vi "IMAQ FPGA Image Transfer to Target U8.vi"(6 "Image Transfer Size Alignment":u32(ring)=1 items=["1 Pixel"=1, "8 Pixels"=8], 7 "Write Timeout (ms)":i32=5000, 8 "error in (no error)":errorcluster, 9 "DMA FIFO Reference In":refnum<k20>, 10 "Maximum Pixels per Write":i32=-1, 11 "Image":T1) -> (0 "error out":errorcluster, 1 "DMA FIFO Reference Out":refnum<k20>, 3 "Image Out":T1)   [LabVIEW 2020, in "NI_VDM_FPGA_Basics.lvlib"]
doc: "Transfers an image from the host processor to the target FPGA via a DMA FIFO."
uses:
  <vilib>/visionFPGA/NI_VDM_FPGA_Basics.lvlib
  <vilib>/vision/Image Controls.llb/IMAQ Image.ctl
  <vilib>/rvi/errors/niLvFpgaAdjustHostInterfaceError.vi
  <vilib>/rvi/interface/nirviMethod/nirviMethod.xnode
  <vilib>/vision/EDVR.llb/IMAQ ImageToEDVR 2D U8.vi
  <vilib>/rvi/errors/niLvFpgaMergeErrorWithErrorCode.vi
  <vilib>/FPGAPlugInAG/Dynamic/niLvFpga_AcquireWriteRegionFifo_Dynamic.vi
  <vilib>/FPGAPlugInAG/Dynamic/niLvFpga_WriteFifo_Dynamic.vi
  nivissvc.dll
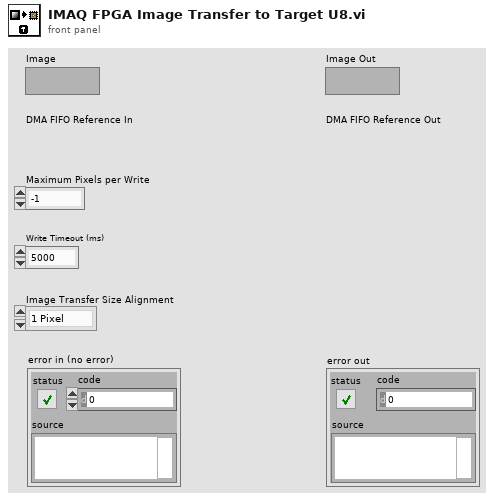
[diagram p1: front panel]
types:
  T1 = typedef "IMAQ Image.ctl" = refnum<image>
  T2 = typedef "Image Type" = u32
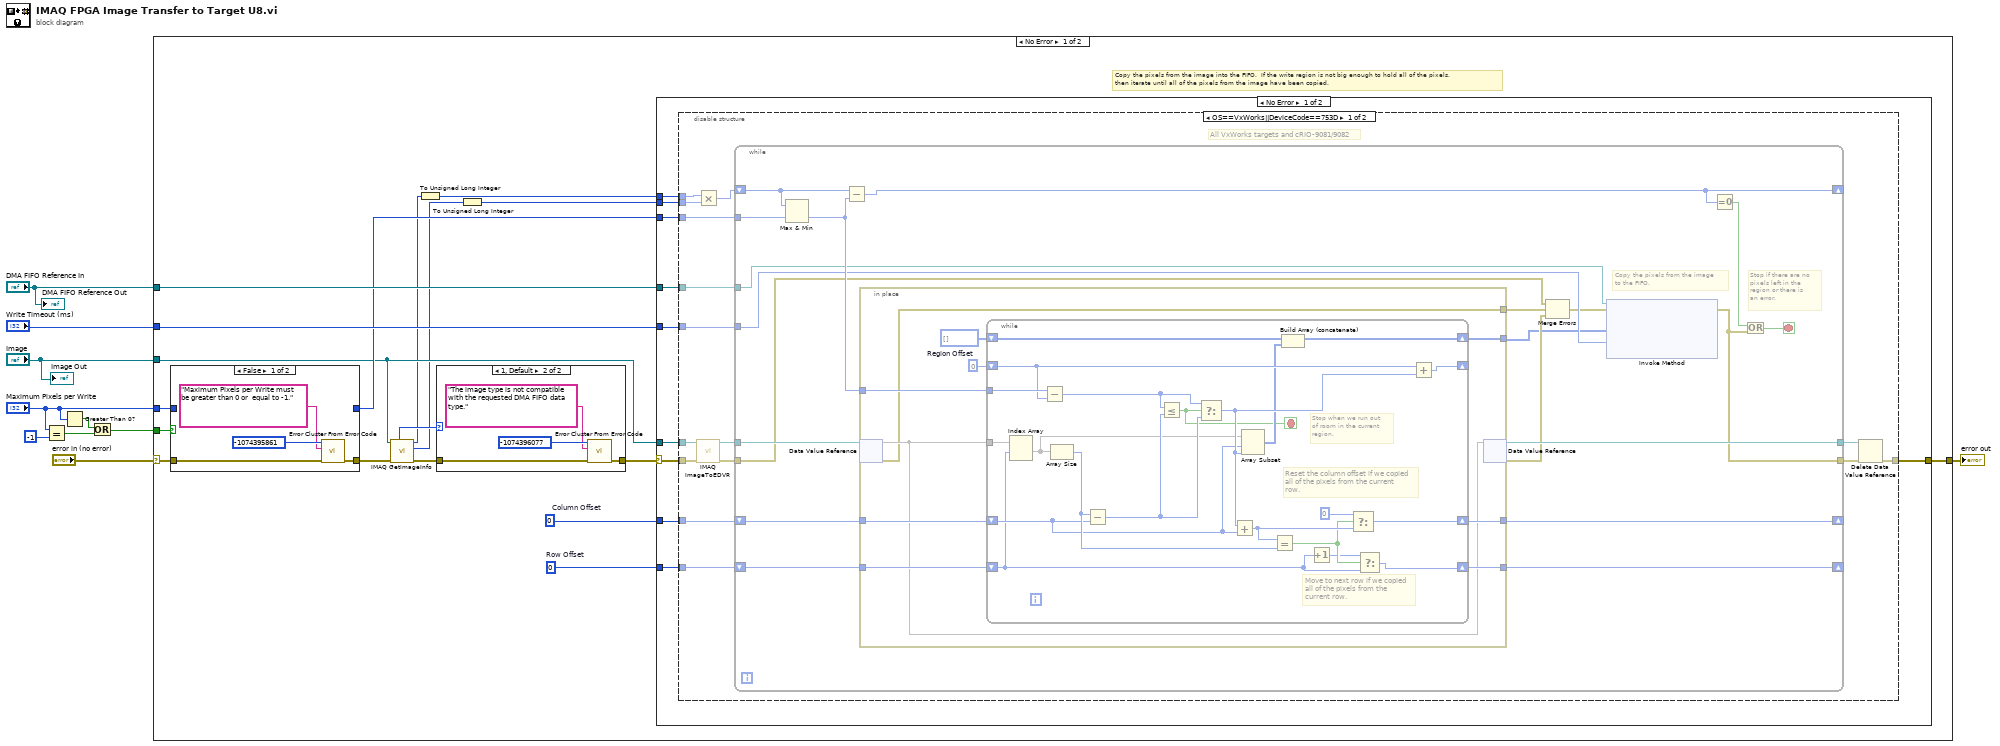
[diagram p0: block diagram]
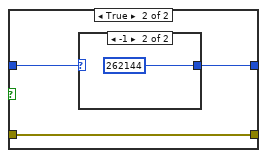
[diagram p2: hidden frame]
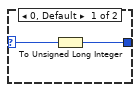
[diagram p3: hidden frame]
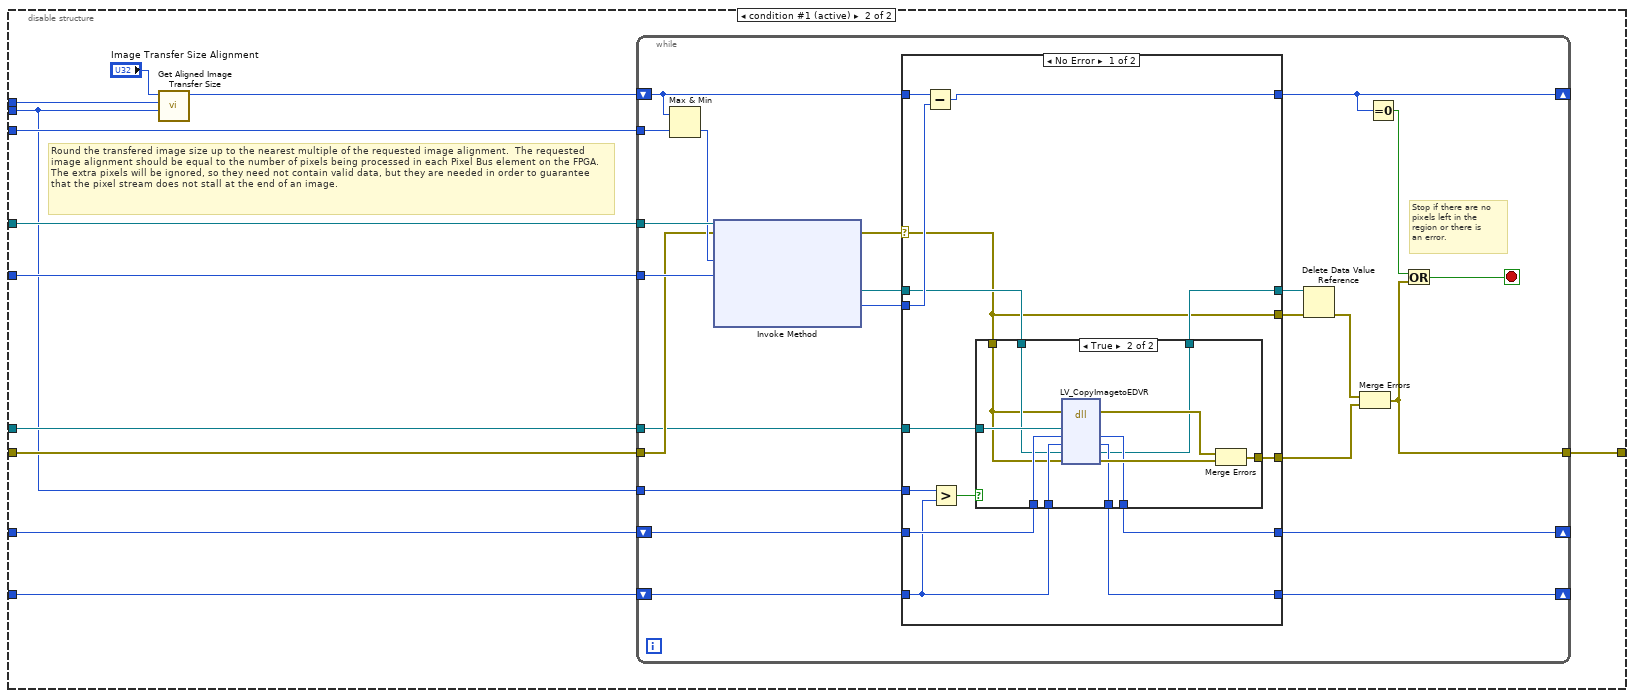
[diagram p4: hidden frame]
diagram:
  n1 = Equal?(x="Maximum Pixels per Write", y=-1) -> (x = y?=w6:bool)
  n2 = Greater Than 0?(x="Maximum Pixels per Write") -> (x > 0?=w7:bool)
  n3 = Or(x=w7, y=w6) -> (x .or. y?=w5:bool)
  n4 = case shown="No Error" "error in (no error)" {
    selector: "error in (no error)" -> [w15 w190]
    tunnel: "DMA FIFO Reference In" -> [w26 _]
    tunnel: "Write Timeout (ms)" -> [w25 _]
    tunnel: w5 -> [w22 _]
    tunnel: "Maximum Pixels per Write" -> [w19 _]
    tunnel: "Image" -> [w17 _]
    tunnel: [w16 w190] -> w2
    frame No Error {
      w23 = u32 0  # Row Offset
      w24 = u32 0  # Column Offset
      # "Copy the pixels from the image into the FIFO.  If the write region is not big enough to hold all of the pixels,\nthen iterate until all of the pixels from the image have been copied."
      n5 = case shown="False" w22 {
        tunnel: w15 -> [w30 w35]
        tunnel: [w29 w35] -> w21
        tunnel: w19 -> [_ w34]
        tunnel: [_ w33] -> w20
        frame False {
          n6 = call <vilib>:"Error Cluster From Error Code.vi"("error in (no error)"=w30, "error message (\"\")"="Maximum Pixels per Write must be greater than 0 or  equal to -1." ("error message (\"\")"), "error code (0)"=-1074395861) -> ("error out"=w29:errorcluster)  [unwired: 6 in]
        }
        frame True {
          n7 = case shown="-1" w34 {
            selector: w34 -> [w37 _]
            tunnel: [w36 u32 262144 ("Maximum Pixels per Write")] -> w33
            frame 0, Default {
              n8 = To Unsigned Long Integer(number=w37) -> (unsigned 32bit integer=w36:u32)
            }
            frame -1 {
            }
          }
        }
      }
      n9 = call "IMAQ GetImageInfo"("error in (no error)"=w21, "Image"=w17) -> ("error out"=w27:errorcluster, "Y Resolution"=w13:i32, "X Resolution"=w14:i32, "Image Type"=w28:T2)  [unwired: 2 in, 4 out]
      n10 = To Unsigned Long Integer(number=w14) -> (unsigned 32bit integer=w12:u32)
      n11 = case shown="1, Default" w28 {
        tunnel: w27 -> [w185 w187]
        tunnel: [w185 w186] -> w18
        frame 0 {
          # "Allowed types are:\nGrayscale (U8)"
        }
        frame 1, Default {
          n12 = call <vilib>:"Error Cluster From Error Code.vi"("error in (no error)"=w187, "error message (\"\")"="The image type is not compatible with the requested DMA FIFO data type." ("error message (\"\")"), "error code (0)"=-1074396077) -> ("error out"=w186:errorcluster)  [unwired: 6 in]
        }
      }
      n13 = To Unsigned Long Integer(number=w13) -> (unsigned 32bit integer=w11:u32)
      n14 = case shown="No Error" w18 {
        selector: w18 -> [w43 w184]
        tunnel: w24 -> [w45 _]
        tunnel: w23 -> [w44 _]
        tunnel: w26 -> [w47 _]
        tunnel: [w41 w184] -> w16
        tunnel: w20 -> [w48 _]
        tunnel: w25 -> [w46 _]
        tunnel: w17 -> [w42 _]
        tunnel: w12 -> [w40 _]
        tunnel: w11 -> [w39 _]
        frame No Error {
          n15 = disable-structure shown="OS==VxWorks||DeviceCode==753D" {
            disable-tunnel: w45 -> [w63 w126]
            disable-tunnel: w44 -> [w62 w125]
            disable-tunnel: w47 -> [w61 w124]
            disable-tunnel: [w52 w123] -> w41
            disable-tunnel: w48 -> [w60 w122]
            disable-tunnel: w46 -> [w59 w121]
            disable-tunnel: w43 -> [w57 w120]
            disable-tunnel: w42 -> [w58 w119]
            disable-tunnel: w40 -> [w51 w116]
            disable-tunnel: w39 -> [w50 w115]
            frame condition #0 {
              # "All VxWorks targets and cRIO-9081/9082"
              n16 = call-poly <vilib>:"IMAQ ImageToEDVR.vi"("error in (no error)"=w57, "Image"=w58) -> ("error out"=w55:errorcluster, "EDVR 2D U8"=w56:refnum<data-value>)  [unwired: 7 in, 1 out]
              n17 = Multiply(x=w51, y=w50) -> (x*y=w49:u32)
              n18 = while {
                shift-right: [w77] -> _
                shift-left: w49 -> [w74]
                tunnel: w56 -> [w83]
                shift-right: [w79] -> _
                shift-left: w63 -> [w81]
                shift-right: [w82] -> _
                shift-left: w62 -> [w80]
                tunnel: w61 -> [w68]
                tunnel: [w78] -> w54
                tunnel: [w66] -> w53
                tunnel: w60 -> [w73]
                tunnel: w59 -> [w69]
                tunnel: w55 -> [w64]
                stop <- w76 stop-if-true
                # "Copy the pixels from the image\nto the FIFO."
                # "Stop if there are no\npixels left in the \nregion or there is\nan error."
                n19 = Max & Min(x=w74, y=w73) -> (min(x,y)=w72:u32)  [unwired: 1 out]
                n20 = Subtract(x=w74, y=w72) -> (x-y=w77:u32)
                n21 = in-place {
                  in-place-border: w72 -> [w91]
                  in-place-border: [w93] -> w82
                  in-place-border: w81 -> [w90]
                  in-place-border: w80 -> [w88]
                  in-place-border: [w89] -> w79
                  in-place-border: [w85] -> w71
                  in-place-border: [w84] -> w65
                  w92 = u32 0  # Region Offset
                  n22 = in-place-dvr #1(w83) -> (w87:u8[][], w85:errorcluster)
                  n23 = while {
                    tunnel: w87 -> [w100]
                    shift-right: [w112] -> _
                    shift-left: w92 -> [w111]
                    tunnel: w91 -> [w114]
                    shift-right: [w105] -> w89
                    shift-left: w90 -> [w101]
                    shift-right: [w95] -> w84
                    shift-left: u8[] [] -> [w97]
                    shift-right: [w102] -> w93
                    shift-left: w88 -> [w98]
                    stop <- w94 stop-if-true
                    # "Stop when we run out\nof room in the current\nregion."
                    # "Reset the column offset if we copied\nall of the pixels from the current\nrow."
                    # "Move to next row if we copied\nall of the pixels from the\ncurrent row."
                    n24 = Index Array(array=w100, index (row)=w98) -> (element=w99:u8[])  [unwired: 1 in]
                    n25 = Subtract(x=w114, y=w111) -> (x-y=w113:u32)
                    n26 = Array Size(array=w99) -> (size(s)=w110:i32)
                    n27 = Subtract(x=w110, y=w101) -> (x-y=w108:u32)
                    n28 = Less Or Equal?(x=w113, y=w108) -> (x <= y?=w94:bool)
                    n29 = Select(t=w113, s=w94, f=w108) -> (s? t:f=w109:u32)
                    n30 = Add(x=w109, y=w101) -> (x+y=w106:u32)
                    n31 = Array Subset(array=w99, index=w101, length=w109) -> (w96:u8[])
                    n32 = Equal?(x=w106, y=w110) -> (x = y?=w104:bool)
                    n33 = Build Array (concatenate)(w97, w96) -> (w95:u8[])
                    n34 = Increment(x=w98) -> (x+1=w103:u32)
                    n35 = Select(t=u32 0 ("Elements In Region"), s=w104, f=w106) -> (s? t:f=w105:u32)
                    n36 = Select(t=w103, s=w104, f=w98) -> (s? t:f=w102:u32)
                    n37 = Add(x=w111, y=w109) -> (x+y=w112:u32)
                  }
                  n38 = in-place-dvr #1(w87) -> (w78:refnum<data-value>, w70:errorcluster)
                }
                n39 = Merge Errors(w64, w71, w70) -> (w67:errorcluster)
                n40 = xnode "Invoke Method"("FPGA VI Reference In"=w68, "error in"=w67, "Data"=w65, "Timeout (ms)"=w69) -> ("error out"=w66:errorcluster)  [unwired: 2 out]
                n41 = Equal To 0?(x=w77) -> (x = 0?=w75:bool)
                n42 = Or(x=w75, y=w66) -> (x .or. y?=w76:bool)
              }
              n43 = Delete Data Value Reference(data value reference=w54, error in=w53) -> (error out=w52:errorcluster)  [unwired: 1 out]
            }
            frame condition #1 (active) {
              # "Round the transfered image size up to the nearest multiple of the requested image alignment.  The requested image alignment should be equal to the number of pixels being processed in each Pixel Bus element on the FPGA.The extra pixels will be ignored, so they need not contain valid data, but they are needed in order to guarantee that the pixel stream does not stall at the end of an image."
              n44 = call <vilib>:"Get Aligned Image Transfer Size.vi"("Y Resolution"=w115, "X Resolution"=w116, "Image Transfer Size Alignment"="Image Transfer Size Alignment") -> ("Aligned Image Transfer Size"=w117:u64)  [unwired: 8 in]
              n45 = while {
                shift-right: [w137] -> _
                shift-left: w117 -> [w132]
                shift-right: [w144] -> _
                shift-left: w126 -> [w146]
                shift-right: [w147] -> _
                shift-left: w125 -> [w145]
                tunnel: w124 -> [w143]
                tunnel: [w135] -> w123
                tunnel: w122 -> [w131]
                tunnel: w121 -> [w130]
                tunnel: w120 -> [w129]
                tunnel: w119 -> [w128]
                tunnel: w115 -> [w127]
                stop <- w136 stop-if-true
                # "Stop if there are no\npixels left in the \nregion or there is\nan error."
                n46 = Max & Min(x=w132, y=w131) -> (min(x,y)=w133:u64)  [unwired: 1 out]
                n47 = xnode "Invoke Method"("FPGA VI Reference In"=w143, "error in"=w129, "Number of Elements"=w133, "Timeout (ms)"=w130) -> ("error out"=w142:errorcluster, "Write Region Reference"=w149:refnum<data-value>, "Elements In Region"=w148:u32)  [unwired: 2 out]
                n48 = case shown="No Error" w142 {
                  selector: w142 -> [w153 w180]
                  tunnel: w132 -> [w163 w183]
                  tunnel: [w162 w183] -> w137
                  tunnel: w149 -> [w158 w179]
                  tunnel: w148 -> [w161 _]
                  tunnel: [w155 w181] -> w147
                  tunnel: w146 -> [w159 w182]
                  tunnel: w145 -> [w151 w181]
                  tunnel: [w156 w182] -> w144
                  tunnel: [w154 w179] -> w141
                  tunnel: [w153 w180] -> w140
                  tunnel: [w157 _] -> w138
                  tunnel: w128 -> [w160 _]
                  tunnel: w127 -> [w150 _]
                  frame No Error {
                    n49 = Subtract(x=w163, y=w161) -> (x-y=w162:u64)
                    n50 = Greater?(x=w150, y=w151) -> (0:w152:bool)
                    n51 = case shown="True" w152 {
                      tunnel: w160 -> [_ w178]
                      tunnel: w159 -> [w164 w177]
                      tunnel: w151 -> [w165 w176]
                      tunnel: w158 -> [w166 w174]
                      tunnel: [w167 w172] -> w157
                      tunnel: [w164 w171] -> w156
                      tunnel: [w165 w170] -> w155
                      tunnel: [w166 w169] -> w154
                      tunnel: w153 -> [w167 w168]
                      frame False {
                      }
                      frame True {
                        n52 = dll-call lib="nivissvc.*" fn="LV_CopyImagetoEDVR" label="LV_CopyImageToEDVR"(error in=w168, "image"=w178, "xImageOffset"=w177, "yImageOffset"=w176, "EDVR"=w174, "error"=w168) -> (error out=w175:errorcluster, "xImageOffset"=w171:u32, "yImageOffset"=w170:u32, "EDVR"=w169:refnum<data-value>, "error"=w173:errorcluster)  [unwired: 4 in, 1 out]
                        n53 = Merge Errors(w175, w173) -> (w172:errorcluster)
                      }
                    }
                  }
                  frame Error {
                  }
                }
                n54 = Delete Data Value Reference(data value reference=w141, error in=w140) -> (error out=w139:errorcluster)  [unwired: 1 out]
                n55 = Merge Errors(w139, w138) -> (w135:errorcluster)
                n56 = Equal To 0?(x=w137) -> (x = 0?=w134:bool)
                n57 = Or(x=w134, y=w135) -> (x .or. y?=w136:bool)
              }
            }
          }
        }
        frame Error {
        }
      }
    }
    frame Error {
    }
  }
  "error out" <- w2
  "Image Out" <- "Image"
  "DMA FIFO Reference Out" <- "DMA FIFO Reference In"
